vi "DAQ_Load_Cells.vi"() -> ()   [LabVIEW 2020]
doc: "I. Description:\nThis example demonstrates how to continuously acquire data (Waveform) using the DAQ device's internal clock and an analog slope start trigger.\n\nII. Instructions for Running:\n1. Select the physical channel to correspond to where your signal is input on the DAQ device.\n2. Enter the minimum and maximum voltage ranges.\nNote: For better accuracy try to match the Input Ranges to the expected voltage level of the measured signal.\n3. Set the rate of the acquisition. Also set the Samples to Read control. This will determine how many samples are read each time the while loop iterates. This also determines how many points are plotted on the graph each iteration.\nNote: The rate should be at least twice as fast as the maximum frequency component of the signal being acquired.\n4. Set the source of the Analog Slope Start Trigger.\n5. Set the slope and level of desired analog edge condition.\n\nIII. Block Diagram Steps:\n1. Create an analog input voltage channel.\n2. Set the rate for the sample clock. Additionally, define the sample mode to be continuous.\n3. Define the parameters for an Analog Slope Start Trigger.\n4. Call the Start VI to start the acquisition.\n5. Read the waveform data in a loop until the user hits the stop button or an error occurs.\n6. Call the Clear Task VI to clear the Task.\n7. Use the popup dialog box to display an error if any.\n\nIV. I/O Connections Overview:\nMake sure your signal input terminal matches the Physical Channel I/O control. Also, make sure your analog trigger terminal matches the Trigger Source Control. For further connection information, refer to your hardware reference manual."
uses:
  <vilib>/Utility/error.llb/DialogType.ctl
  <vilib>/ULx/Create Channel.llb/ULx Create Channel (AI-Voltage-Basic).vi
  <vilib>/ULx/Timing.llb/ULx Timing (Sample Clock).vi
  <vilib>/ULx/Read.llb/ULx Read (Analog 1D Wfm NChan NSamp).vi
panel:
  in  "stop 2":bool
  in  "maximum value":dbl=5.0
  in  "minimum value":dbl=-5.0
  in  "Physical Channel":refnum<k21>="Dev0/Ai0"
  out "Measurement":waveform(dbl)[](graph)
  # "For instructions, select Help>>Show Context Help"
  # "Channel Parameters"
  # "* Please refer to your device documentation for information \nregarding valid Analog Triggers for your device."
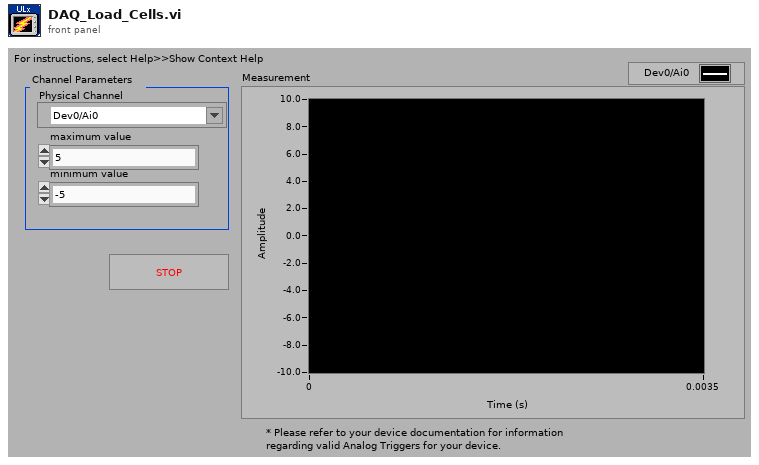
[diagram p1: front panel]
types:
  T1 = typedef "DialogType.ctl" = u16
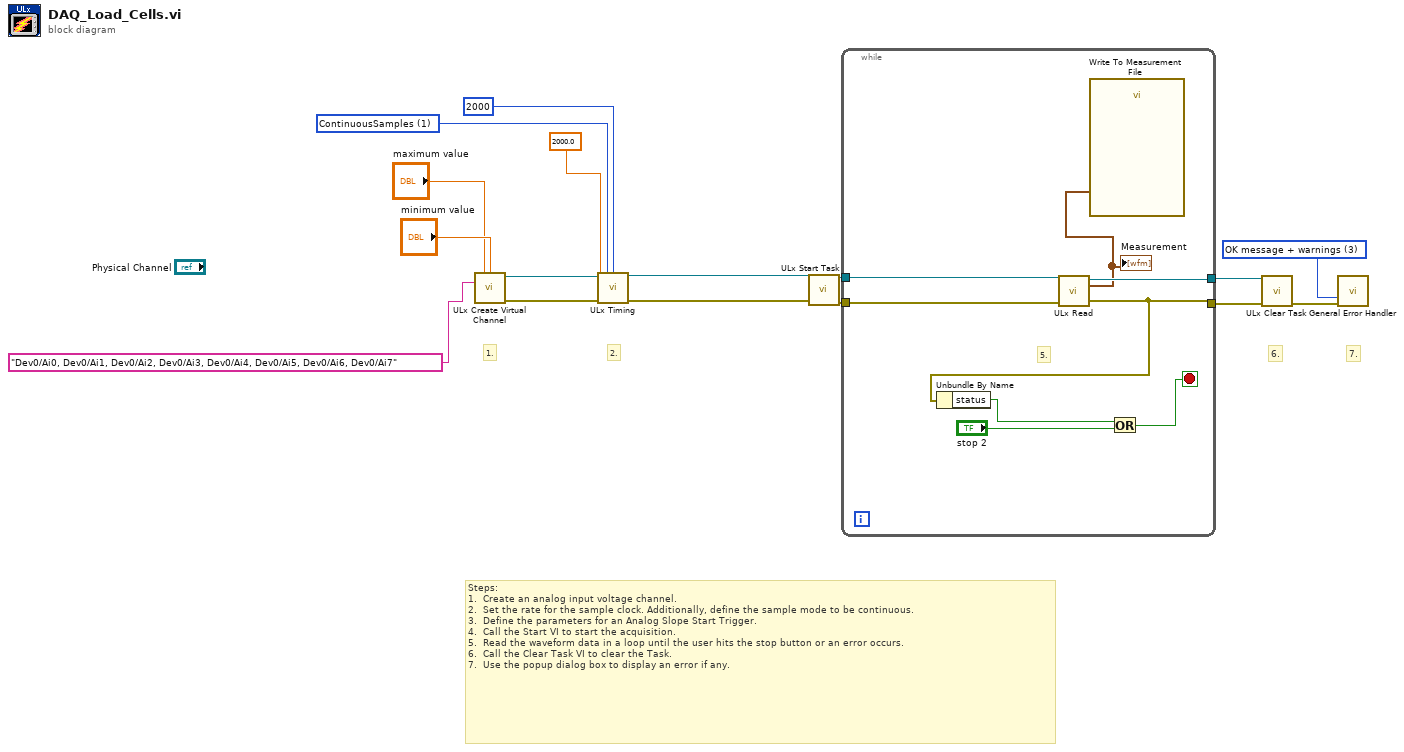
[diagram p0: block diagram]
diagram:
  w2 = 1 items=["FiniteSamples", "ContinuousSamples"] ("sample mode")
  w9 = T1 3 items=["no dialog", "OK message", "continue or stop message", "OK message + warnings", "continue/stop + warnings"] ("type of dialog (OK msg:1)")
  # "7."
  # "6."
  # "Steps: \n1.  Create an analog input voltage channel.\n2.  Set the rate for the sample clock. Additionally, define the sample mode to be continuous.\n3.  Define the parameters for an Analog Slope Start Trigger.\n4.  Call the Start VI to start the acquisition.\n5.  Read the waveform data in a loop until the user hits the stop button or an error occurs.\n6.  Call the Clear Task VI to clear the Task.\n7.  Use the popup dialog box to display an error if any."
  # "2."
  # "1."
  n1 = call-poly <vilib>:"ULx Create Virtual Channel.vi"("maximum value"="maximum value", "minimum value"="minimum value", "physical channels"="Dev0/Ai0, Dev0/Ai1, Dev0/Ai2, Dev0/Ai3, Dev0/Ai4, Dev0/Ai5, Dev0/Ai6, Dev0/Ai7") -> ("task out"=w13:refnum<k24>, "error out"=w16:errorcluster)  [unwired: 11 in]
  n2 = call-poly <vilib>:"ULx Timing.vi"("task in"=w13, "sample mode"=w2, "samples per channel"=2000, "rate"=2000.0, "error in"=w16) -> ("task out"=w8:refnum<k24>, "error out"=w7:errorcluster)  [unwired: 9 in]
  n3 = call <vilib>:"ULx Start Task.vi"("task in"=w8, "error in"=w7) -> ("task out"=w12:refnum<k24>, "error out"=w15:errorcluster)  [unwired: 12 in]
  n4 = while {
    tunnel: w15 -> [w24]
    tunnel: w12 -> [w23]
    tunnel: [w22] -> w11
    tunnel: [w18] -> w10
    stop <- w17 stop-if-true
    # "5."
    n5 = call-poly <vilib>:"ULx Read.vi"("task in"=w23, "error in"=w24) -> ("task out"=w22:refnum<k24>, "data"=w21:waveform(dbl)[], "error out"=w18:errorcluster)  [unwired: 11 in]
    "Measurement" <- w21
    n6 = Unbundle By Name(w18) -> ("status"=w20:bool)
    n7 = call "Write To Measurement File"("Signals"=w21) -> ()  [unwired: 16 in, 3 out]
    n8 = Or(x=w20, y="stop 2") -> (x .or. y?=w17:bool)
  }
  n9 = call <vilib>:"ULx Clear Task.vi"("task in"=w11, "error in"=w10) -> ("error out"=w14:errorcluster)  [unwired: 13 in]
  n10 = call <vilib>:"General Error Handler.vi"("type of dialog (OK msg:1)"=w9, "error in (no error)"=w14) -> ()  [unwired: 9 in, 5 out]
